vi "Submit Channel Config.vi"(8 "error in (no error)":errorcluster, 10 "Asset Name":string, 11 "Sift Client in":refnum<class "Sift Client.lvclass">) -> (0 "error out":errorcluster, 3 "Sift Client out":refnum<class "Sift Client.lvclass">)   [LabVIEW 2024, in "Sift Client.lvlib" / "Sift Client.lvclass"]
uses:
  Sift Client.lvclass
  Private/Typedefs/Ingestion Config.ctl
  Private/Typedefs/Flow Config.ctl
  Private/Typedefs/Channel Config.ctl
  Types/Data Type.ctl
  Private/Typedefs/Bit Field.ctl
  Private/Typedefs/Enum.ctl
  Sift Client.lvclass/Sift Client.ctl
  <vilib>/addons/_JKI.lib/Serialization/JSON/JKI JSON Serialization.lvlib
  Sift Client.lvlib
panel:
  in  "Ingestion Config":T1
  out "JSON String":string
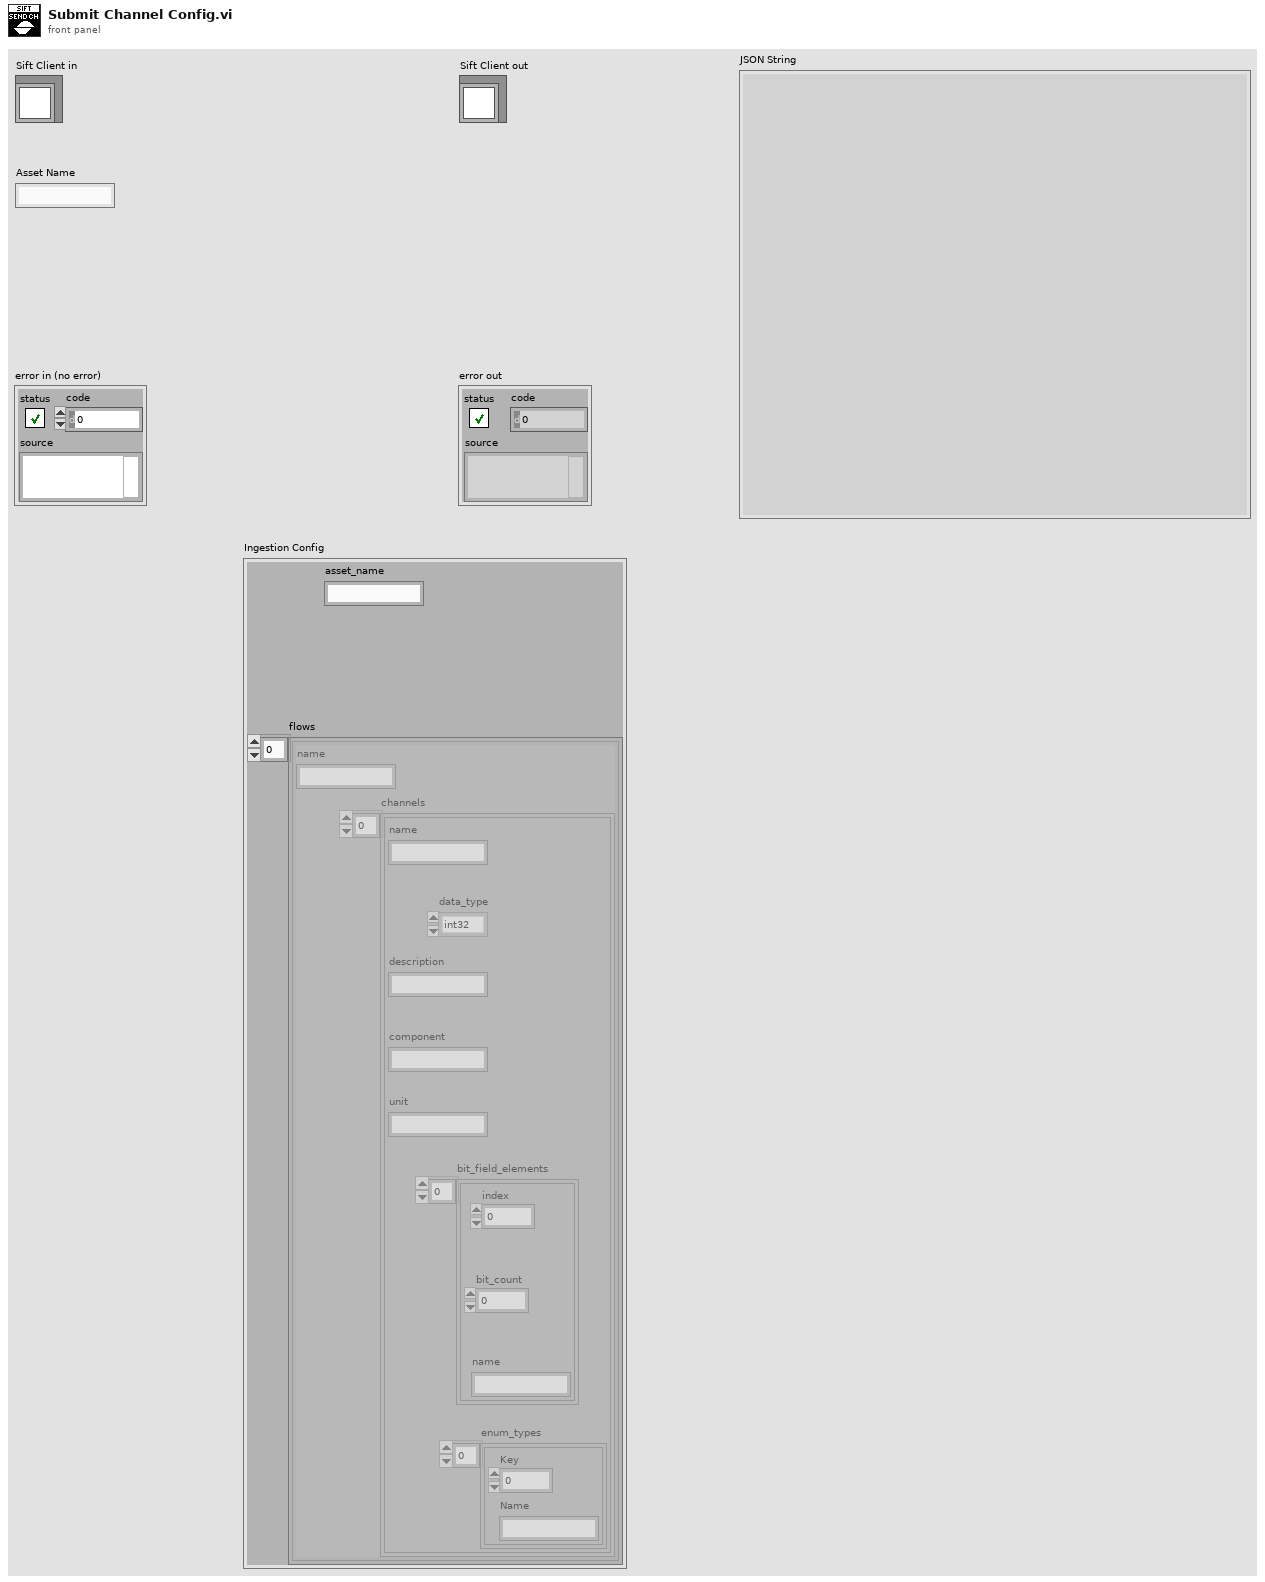
[diagram p1: front panel]
types:
  T1 = typedef "Sift Client.lvlib/Ingestion Config.ctl" = cluster{"asset_name":string, "flows":T2[]}
  T2 = typedef "Sift Client.lvlib/Flow Config.ctl" = cluster{"name":string, "channels":T3[]}
  T3 = typedef "Sift Client.lvlib/Channel Config.ctl" = cluster{"name":string, "data_type":T4, "description":string, "component":string, "unit":string, "bit_field_elements":T5[], "enum_types":T6[]}
  T4 = typedef "Sift Client.lvlib/Data Type.ctl" = enum8{"double", "float", "uint64", "int64", "uint32", "int32", "bool", "bit field", "enum"}
  T5 = typedef "Sift Client.lvlib/Bit Field.ctl" = cluster{"index":u32, "bit_count":u32, "name":string}
  T6 = typedef "Sift Client.lvlib/Enum.ctl" = cluster{"Key":u32, "Name":string}
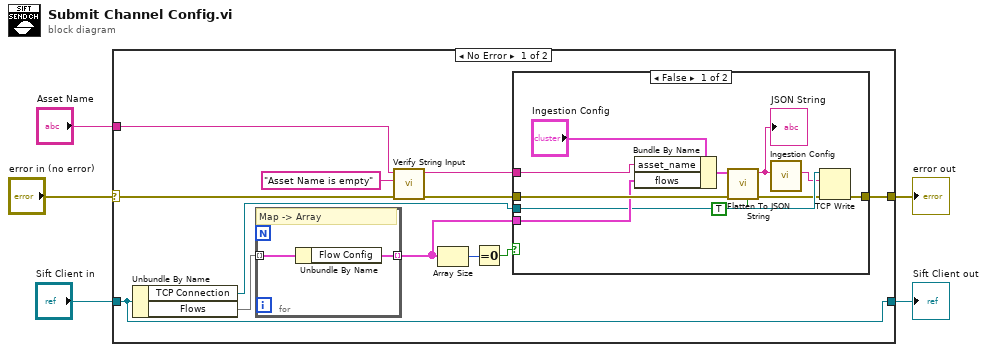
[diagram p0: block diagram]
diagram:
  n1 = case shown="No Error" "error in (no error)" {
    selector: "error in (no error)" -> [w12 w33]
    tunnel: [w16 w33] -> w4
    tunnel: [w15 w32] -> w2
    tunnel: "Sift Client in" -> [w15 w32]
    tunnel: "Asset Name" -> [w14 _]
    frame No Error {
      n2 = Unbundle By Name(w15) -> ("TCP Connection"=w17:refnum<k5>, "Flows"=w9:map{string, T2})
      n3 = for {
        tunnel: [w18] -> w8 mode=indexing
        tunnel: w9 -> [w19] mode=indexing
        # "Map -> Array"
        n4 = Unbundle By Name(w19) -> ("Flow Config"=w18:T2)
      }
      n5 = call "Verify String Input.vi"("error in (no error)"=w12, "Error Message"="Asset Name is empty", "Input"=w14) -> ("error out"=w11:errorcluster, "Output"=w10:string)  [unwired: 7 in]
      n6 = Array Size(array=w8) -> (size(s)=w7:i32)
      n7 = Equal To 0?(x=w7) -> (x = 0?=w6:bool)
      n8 = case shown="False" w6 {
        tunnel: w10 -> [w28 _]
        tunnel: w17 -> [w24 _]
        tunnel: w11 -> [w30 w31]
        tunnel: [w21 w31] -> w16
        tunnel: w8 -> [w27 _]
        frame False {
          n9 = Bundle By Name(cluster="Ingestion Config", "asset_name"=w28, "flows"=w27) -> (w26:T1)
          n10 = call <vilib>:"Flatten To JSON String.vi"("Enums As String (F)"=TRUE, "error in"=w30, "Variant"=w26) -> ("error out"=w22:errorcluster, "JSON String"=w25:string)  [unwired: 7 in]
          "JSON String" <- w25
          n11 = call "Ingestion Config.vi"("Data"=w25) -> ("Message"=w23:string)  [unwired: 10 in]
          n12 = TCP Write(connection ID=w24, data in=w23, error in (no error)=w22) -> (error out=w21:errorcluster)  [unwired: 1 in, 2 out]
        }
        frame True {
        }
      }
    }
    frame Error {
    }
  }
  "error out" <- w4
  "Sift Client out" <- w2
